vi "Periodic Tasks.vi"(8 "error in":errorcluster) -> ()   [LabVIEW 2015]
doc: "This VI runs in parallel to other tasks. It can contain as many user-defined periodic loops as you need. These can carry out PID or other sorts of timed response."
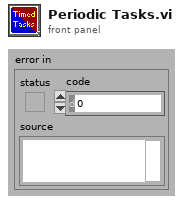
[diagram p1: front panel]
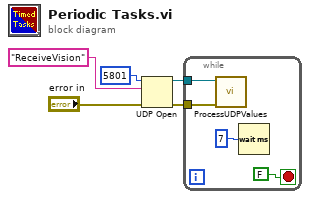
[diagram p0: block diagram]
diagram:
  n1 = UDP Open(8:"error in", 10:"ReceiveVision" ("service name"), 11:u16 5801 ("port")) -> (port=w3:refnum<k16>, 0:w2:errorcluster)  [unwired: 2 in, 1 out]
  n2 = while {
    tunnel: w3 -> [w7]
    tunnel: w2 -> [w6]
    stop <- FALSE stop-if-true
    n3 = call "ProcessUDPValues.vi"("error in (no error)"=w6, "connection ID"=w7) -> ()  [unwired: 10 in]
    n4 = Wait (ms)(milliseconds to wait=u32 7) -> ()  [unwired: 1 out]
  }
